vi "demo.vi"() -> ()   [LabVIEW 2012, in "FileSystem Watcher.lvlib"]
uses:
  FileSystem Watcher.lvlib
panel:
  out "错误输出":errorcluster
  in  "filter":string
  in  "Dir Path":path
  in  "停止按钮":bool
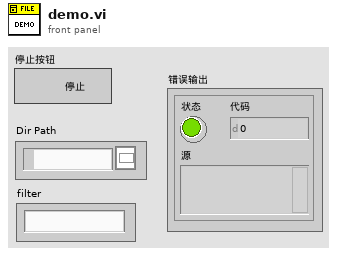
[diagram p1: front panel]
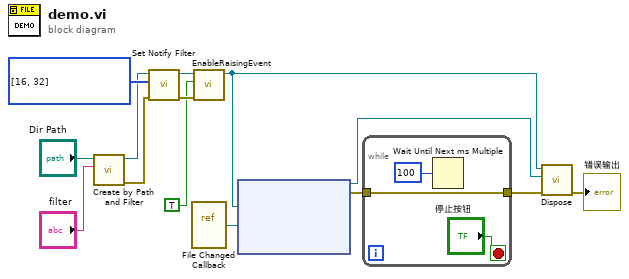
[diagram p0: block diagram]
diagram:
  w9 = i32[] [16, 32] items=["FileName"=1, "DirectoryName"=2, "Attributes"=4, "Size"=8, "LastWrite"=16, "LastAccess"=32, "CreationTime"=64, "Security"=256] ("Notify Filter")
  n1 = call "Create by Path and Filter.vi"("filter"="filter", "Dir Path"="Dir Path") -> ("错误输出"=w10:errorcluster, "FileSystem Watcher Ref"=w8:refnum<k24>)  [unwired: 8 in]
  n2 = call "Set Notify Filter.vi"("错误输入（无错误）"=w10, "Notify Filter"=w9, "FilesytemWatcher Ref In"=w8) -> ("错误输出"=w6:errorcluster, "FilesytemWatcher Ref Out"=w7:refnum<k24>)  [unwired: 7 in]
  n3 = vi-ref "File Changed Callback.vi"() -> ("vi reference"=w14:refnum<vi>)
  n4 = call "EnableRaisingEvent.vi"("错误输入（无错误）"=w6, "EnableRaisingEvents"=TRUE, "FilesytemWatcher Ref In"=w7) -> ("FilesytemWatcher Ref Out"=w3:refnum<k24>)  [unwired: 7 in, 1 out]
  n5 = node(w3, w14) -> (w2:refnum<k27>, w13:errorcluster)  [unwired: 3 in]
  n6 = while {
    tunnel: w13 -> [w15]
    tunnel: [w15] -> w4
    stop <- "停止按钮" stop-if-true
    n7 = Wait Until Next ms Multiple(millisecond multiple=u32 100 ("毫秒倍数")) -> ()  [unwired: 1 out]
  }
  n8 = call "Dispose.vi"("错误输入（无错误）"=w4, "事件注册引用句柄"=w2, "Filesytem Watcher Ref"=w3) -> ("错误输出"=→"错误输出":errorcluster)  [unwired: 8 in]
